vi "Error Reporter.vi"(9 "Status Value":u16 format="%04x", 10 "Status Number":u8=61, 11 "Command":T1(ring)=enum."Set Statuses") -> ()   [LabVIEW 2014]
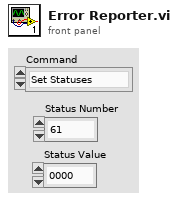
[diagram p1: front panel]
types:
  T1 = enum16{"Default", "Set Statuses", "Set Parameters", "Save Parameter"}
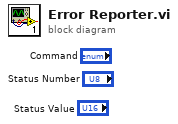
[diagram p0: block diagram]
diagram:
